vi "Print IntGraph.vi"(1 "Data IntGraph":dbl[][](graph)) -> ()   [LabVIEW 2020]
uses:
  Instance           1 22Saved   Print IntGraph .vi
panel:
  out "String":string
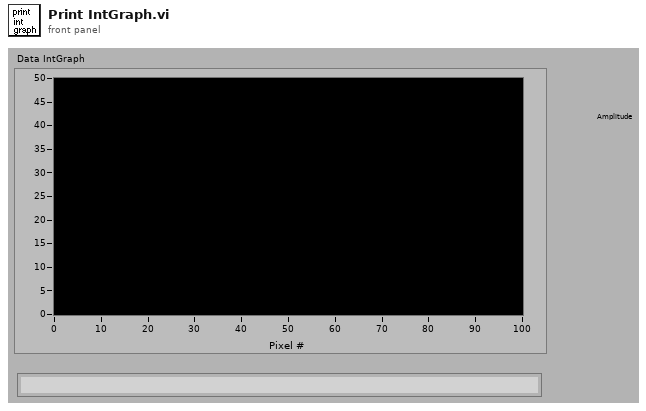
[diagram p1: front panel]
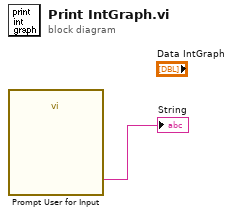
[diagram p0: block diagram]
diagram:
  n1 = call "Prompt User for Input"() -> ("Plot_Info"=→"String":string)  [unwired: 17 in, 2 out]
